vi "DHT11 Reading Data.vi"(8 "Error In":errorcluster) -> (0 "Error Out":errorcluster)   [LabVIEW 2014, in "ESP8266 WiFi Wrapper.lvlib"]
uses:
  <vilib>/Aledyne-TSXperts/Arduino Compatible Compiler for LabVIEW/addons/ESP8266 WiFi Wrapper/ESP8266 WiFi Wrapper.lvlib
  <vilib>/Aledyne-TSXperts/Arduino Compatible Compiler for LabVIEW/Arduino Compatible Compiler for LabVIEW.lvlib
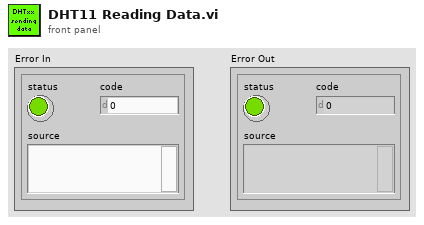
[diagram p1: front panel]
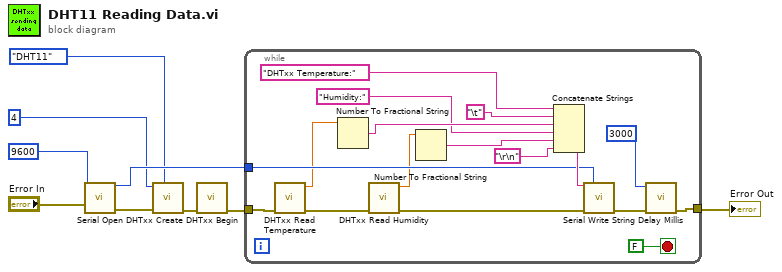
[diagram p0: block diagram]
diagram:
  n1 = call <vilib>:"Serial Open.vi"("Speed"=u32 9600, "error in (no error)"="Error In") -> ("Instance"=w7:u8, "error out"=w5:errorcluster)  [unwired: 12 in]
  n2 = call <vilib>:"DHTxx Create.vi"("DHT Type"=enum16{"DHT11", "DHT21", "DHT22"}."DHT11", "Error In"=w5, "DHT pin"=u8 4) -> ("Error Out"=w2:errorcluster)  [unwired: 8 in]
  n3 = call <vilib>:"DHTxx Begin.vi"("Error In"=w2) -> ("Error Out"=w1:errorcluster)  [unwired: 10 in]
  n4 = while {
    tunnel: [w25] -> w8
    tunnel: w7 -> [w21]
    tunnel: w1 -> [w20]
    stop <- FALSE stop-if-true
    n5 = call <vilib>:"DHTxx Read Temperature.vi"("Error In"=w20) -> ("Error Out"=w15:errorcluster, "Temperature"=w18:dbl)  [unwired: 9 in]
    n6 = Number To Fractional String(number=w18) -> (F-format string=w19:string)  [unwired: 3 in]
    n7 = call <vilib>:"DHTxx Read Humidity.vi"("Error In"=w15) -> ("Error Out"=w16:errorcluster, "Humidity"=w17:dbl)  [unwired: 9 in]
    n8 = Number To Fractional String(number=w17) -> (F-format string=w14:string)  [unwired: 3 in]
    n9 = Concatenate Strings("DHTxx Temperature:" ("string"), "\t" ("Tab Constant"), w19, "Humidity:" ("string"), w14, "\r\n" ("End of Line Constant")) -> (w22:string)
    n10 = call <vilib>:"Serial Write String.vi"("String"=w22, "Instance"=w21, "error in (no error)"=w16) -> ("error out"=w26:errorcluster)  [unwired: 12 in]
    n11 = call <vilib>:"Delay Millis.vi"("error in (no error)"=w26, "delay"=u32 3000) -> ("error out"=w25:errorcluster)  [unwired: 9 in]
  }
  "Error Out" <- w8
